vi "OpenMUXRelay.vi"(8 "error in (no error)":errorcluster, 10 "gRPCid":T2, 11 "ctet_mux in":T1) -> (0 "error out":errorcluster, 3 "ctet_mux out":T1)   [LabVIEW 2019, in "ctet_mux_User Library.lvlib"]
uses:
  ctet_mux_User Library.lvlib
  Servers/ctet_mux/gRPC lvSupport/Server API/typeDefs/grpcId.ctl
  Types/ctet_mux.ctl
  <instrlib>/niSwitch/niSwitch.llb/niSwitch Relay Action.ctl
  Servers/ctet_mux/ctet_mux Class/RPC Messages/measurementservice_MUXOpenRelayResponse/measurementservice_MUXOpenRelayResponse_Data.ctl
  Servers/ctet_mux/ctet_mux Class/RPC Messages/measurementservice_ErrorOut/measurementservice_ErrorOut_Data.ctl
  Types/Switch Action.ctl
  Servers/ctet_mux/ctet_mux Class/ctet_mux.lvclass
  Servers/ctet_mux/gRPC lvSupport/gprc-lvsupport.lvlib
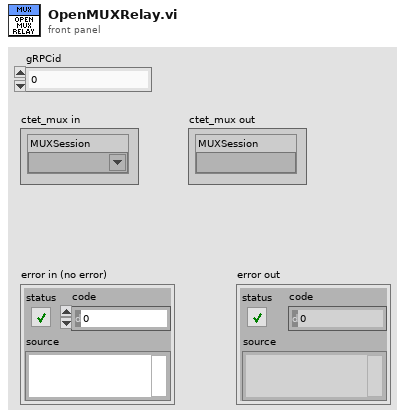
[diagram p1: front panel]
types:
  T1 = typedef "ctet_mux_User Library.lvlib/ctet_mux.ctl" = cluster{"MUXSession":refnum<k15>}
  T2 = typedef "ctet_mux.lvlib/gprc-lvsupport.lvlib/grpcId.ctl" = u64
  T3 = typedef "ctet_mux_User Library.lvlib/Switch Action.ctl" = enum16{"Get Switch State", "Initialize", "Connect Channel", "Open Channel", "Close Relay", "Open Relay", "Disconnect/Open All"}
  T4 = typedef "ctet_mux.lvlib/ctet_mux.lvclass/measurementservice_ErrorOut_Data.ctl" = cluster{"errCode":i64, "errMessage":string}
  T5 = typedef "ctet_mux.lvlib/ctet_mux.lvclass/measurementservice_MUXOpenRelayResponse_Data.ctl" = cluster{"error":T4}
  T6 = typedef "niSwitch Relay Action.ctl" = i32
  T7 = typedef "ctet_mux.lvlib/ctet_mux.lvclass/measurementservice_MUXOpenRelayRequest_Data.ctl" = cluster{"RelayName":string}
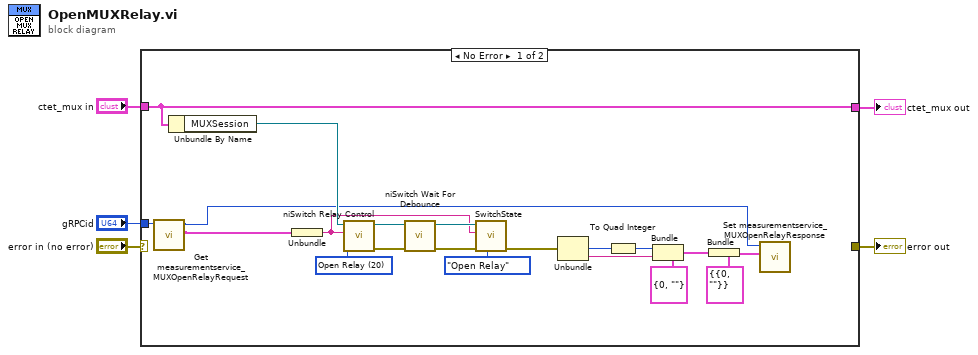
[diagram p0: block diagram]
diagram:
  n1 = case shown="No Error" "error in (no error)" {
    selector: "error in (no error)" -> [_ w27]
    tunnel: [_ w27] -> w5
    tunnel: "gRPCid" -> [w17 _]
    tunnel: "ctet_mux in" -> [w22 w26]
    tunnel: [w22 w26] -> w1
    frame No Error {
      w18 = T6 20 items=["Open Relay"=20, "Close Relay"=21] ("relay action (Close Relay)")
      n2 = call "Get measurementservice_MUXOpenRelayRequest.vi"("gRPCid"=w17) -> ("Message Data"=w16:T7, "gRPCid out"=w13:T2)  [unwired: 8 in, 1 out]
      n3 = Unbundle By Name(w22) -> ("MUXSession"=w19:refnum<k15>)
      n4 = Unbundle(w16) -> ("RelayName"=w7:string)
      n5 = call <instrlib>:"niSwitch Relay Control.vi"("relay action (Close Relay)"=w18, "relay names"=w7, "instrument handle"=w19) -> ("error out"=w20:errorcluster, "instrument handle out"=w21:refnum<k15>)  [unwired: 7 in]
      n6 = call <instrlib>:"niSwitch Wait For Debounce.vi"("error in (no error)"=w20, "instrument handle"=w21) -> ("error out"=w9:errorcluster, "instrument handle out"=w10:refnum<k15>)  [unwired: 8 in]
      n7 = call "SwitchState.vi"("Switch Action"=Switch_Action."Open Relay", "error in (no error)"=w9, "channel 1"=w7, "Switch Session"=w10) -> ("error out"=w8:errorcluster)  [unwired: 5 in, 2 out]
      n8 = Unbundle(w8) -> ("code"=w24:i32, "source"=w25:string)  [unwired: 1 out]
      n9 = To Quad Integer(1:w24) -> (0:w23:i64)
      n10 = Bundle(cluster=T4 {"errCode"=0, "errMessage"=""} ("error"), "errCode"=w23, "errMessage"=w25) -> (w11:T4)
      n11 = Bundle(cluster=T5 {"error"={"errCode"=0, "errMessage"=""}} ("measurementservice_MUXOpenRelayResponse_Data"), "error"=w11) -> (w14:T5)
      n12 = call "Set measurementservice_MUXOpenRelayResponse.vi"("Message Data"=w14, "gRPCid"=w13) -> ()  [unwired: 9 in, 1 out]
    }
    frame Error {
    }
  }
  "error out" <- w5
  "ctet_mux out" <- w1
